vi "7HP_Set serial timeout.vi"(8 "Error In":errorcluster, 10 "timeout (ms)":u32=2000, 11 "VISA resource name":refnum<visa-resource-name>) -> (0 "Error Out":errorcluster, 3 "VISA resource name out":refnum<visa-resource-name>)   [LabVIEW 2017]
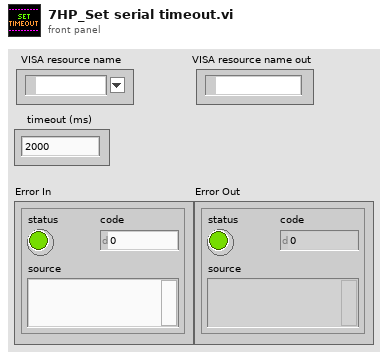
[diagram p1: front panel]
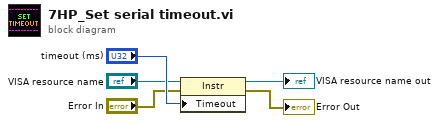
[diagram p0: block diagram]
diagram:
  n1 = property class="Instr"(reference="VISA resource name", error in="Error In", "Timeout"="timeout (ms)") -> (reference out=→"VISA resource name out":refnum<visa-resource-name>, error out=→"Error Out":errorcluster)
